vi "Indexed String To Enum.vi"(7 "Variant":variant, 8 "error in (no error)":errorcluster, 11 "String":string) -> (0 "error out":errorcluster, 3 "Enum":variant)   [LabVIEW 2017]
doc: "Converts a string into an enum value. A leading number selects the entry by index, otherwise the entry is chosen by matching the string content case-insensitively."
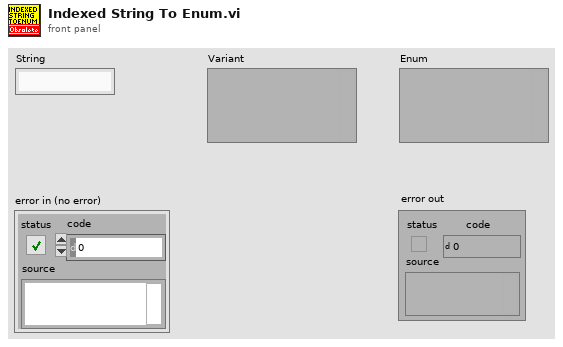
[diagram p1: front panel]
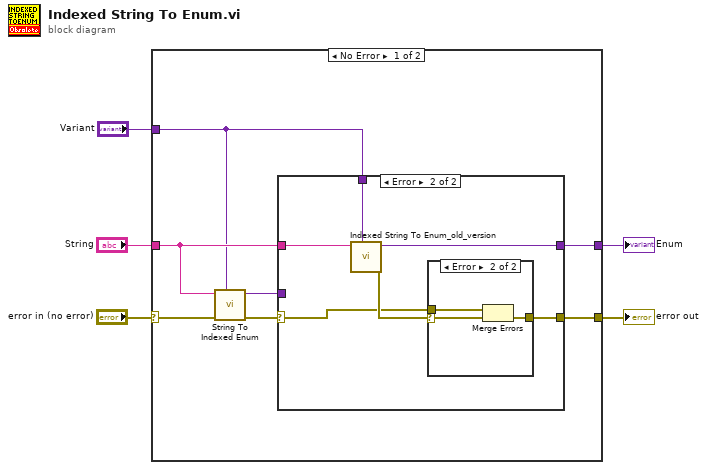
[diagram p0: block diagram]
diagram:
  n1 = case shown="No Error" "error in (no error)" {
    selector: "error in (no error)" -> [w8 w26]
    tunnel: [w12 w26] -> w5
    tunnel: [w11 w25] -> w4
    tunnel: "String" -> [w10 _]
    tunnel: "Variant" -> [w9 w25]
    frame No Error {
      n2 = call "String To Indexed Enum.vi"("Variant"=w9, "error in (no error)"=w8, "String"=w10) -> ("error out"=w7:errorcluster, "Enum"=w6:variant)  [unwired: 7 in]
      n3 = case shown="Error" w7 {
        selector: w7 -> [w13 w15]
        tunnel: [w13 w16] -> w12
        tunnel: [w14 w20] -> w11
        tunnel: w10 -> [_ w19]
        tunnel: w9 -> [_ w18]
        tunnel: w6 -> [w14 _]
        frame No Error {
        }
        frame Error {
          n4 = call "Indexed String To Enum_old_version.vi"("Variant"=w18, "String"=w19) -> ("error out"=w17:errorcluster, "Enum"=w20:variant)  [unwired: 8 in]
          n5 = case shown="Error" w17 {
            selector: w17 -> [w21 w24]
            tunnel: [w21 w23] -> w16
            tunnel: w15 -> [_ w22]
            frame No Error {
            }
            frame Error {
              n6 = Merge Errors(w22, w24) -> (w23:errorcluster)
            }
          }
        }
      }
    }
    frame Error {
    }
  }
  "Enum" <- w4
  "error out" <- w5
